vi "zadanie4.vi"() -> ()   [LabVIEW 2019]
uses:
  <vilib>/Utility/file.llb/Write Delimited Spreadsheet (DBL).vi
  <vilib>/ptbypt/NI_PtbyPt.lvlib
panel:
  out "Histogram":dynamicdata(graph)
  out "XY Graph":cluster{"time":dbl[], "value":dbl[]}(graph)
  out "Waveform Chart":cluster{"Numeric":dbl, "mean":dbl}(graph)
  in  "stop":bool
  out "Numeric":dbl
  out "read buffer":string
  in  "Light intensity [%]":dbl(ramp)
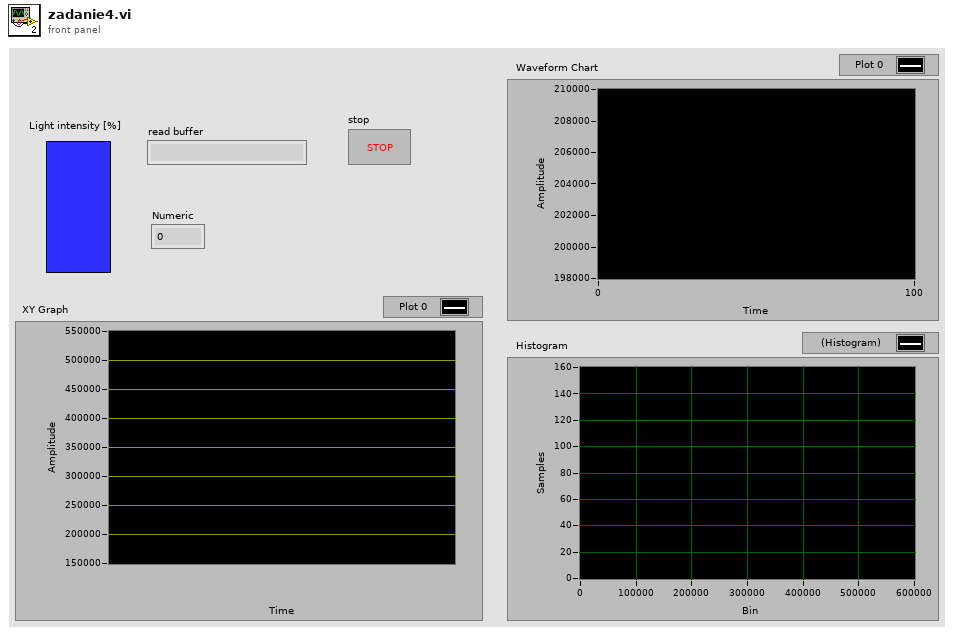
[diagram p1: front panel]
types:
  T1 = enum16{"Configure Port", "Write", "Read", "Close"}
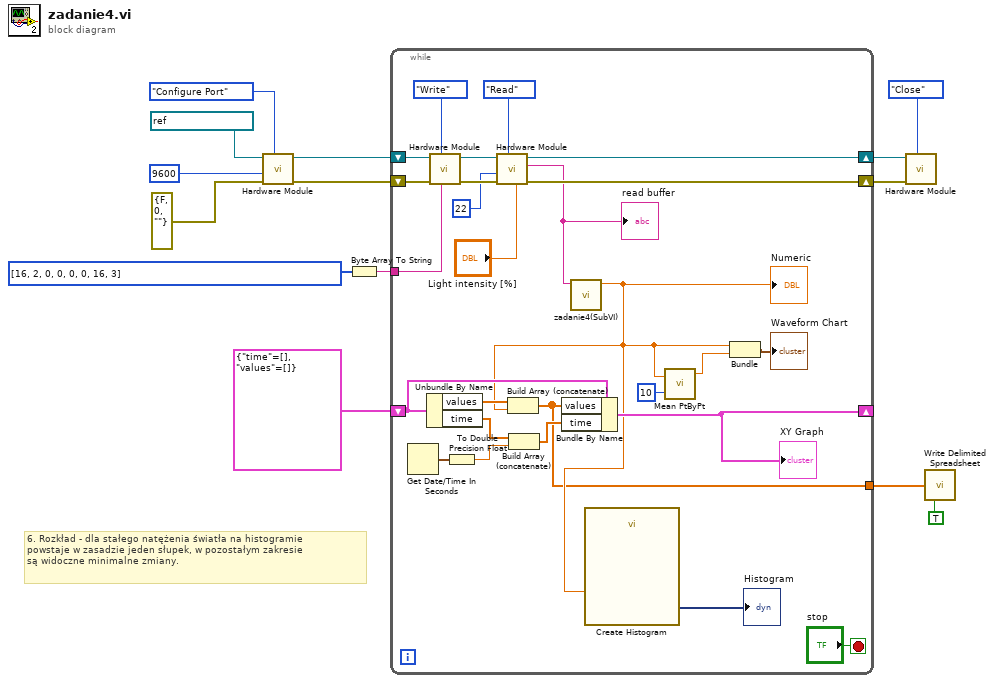
[diagram p0: block diagram]
diagram:
  # "6. Rozkład - dla stałego natężenia światła na histogramie \npowstaje w zasadzie jeden słupek, w pozostałym zakresie \nsą widoczne minimalne zmiany."
  n1 = call "Hardware Module.vi"("State"=T1."Configure Port", "error in (no error)"=errorcluster {"status"=FALSE, "code"=0, "source"=""}, "baud rate (9600)"=u32 9600, "VISA resource name"=refnum<visa-resource-name> "VirtualDevice1") -> ("error out"=w12:errorcluster, "VISA resource name out"=w11:refnum<visa-resource-name>)  [unwired: 4 in, 2 out]
  n2 = Byte Array To String(unsigned byte array=u8[] [16, 2, 0, 0, 0, 0, 16, 3]) -> (string=w4:string)
  n3 = while {
    tunnel: w4 -> [w32]
    shift-right: [w37] -> w13
    shift-left: w12 -> [w36]
    shift-right: [w39] -> w14
    shift-left: w11 -> [w35]
    shift-right: [w21] -> _
    shift-left: cluster{"time":dbl[], "values":dbl[]} {"time"=[], "values"=[]} -> [w27]
    tunnel: [w15] -> w2
    stop <- "stop" stop-if-true
    n4 = Get Date/Time In Seconds() -> (seconds since 1Jan1904=w23:timestamp)
    n5 = Unbundle By Name(w27) -> ("values"=w26:dbl[], "time"=w25:dbl[])
    n6 = call "Hardware Module.vi"("write buffer"=w32, "State"=T1."Write", "error in (no error)"=w36, "VISA resource name"=w35) -> ("error out"=w38:errorcluster, "VISA resource name out"=w40:refnum<visa-resource-name>)  [unwired: 4 in, 2 out]
    n7 = To Double Precision Float(number=w23) -> (double precision float=w22:dbl)
    n8 = call "Hardware Module.vi"("Light intensity [%]"="Light intensity [%]", "State"=T1."Read", "error in (no error)"=w38, "byte count"=u32 22, "VISA resource name"=w40) -> ("error out"=w37:errorcluster, "read buffer"=w29:string, "VISA resource name out"=w39:refnum<visa-resource-name>)  [unwired: 3 in, 1 out]
    "read buffer" <- w29
    n9 = Build Array (concatenate)(w25, w22) -> (w24:dbl[])
    n10 = call "zadanie4(SubVI).vi"("read buffer"=w29) -> ("Numeric"=w17:dbl)  [unwired: 10 in]
    "Numeric" <- w17
    n11 = Build Array (concatenate)(w26, w17) -> (w15:dbl[])
    n12 = Bundle By Name(cluster=w27, "values"=w15, "time"=w24) -> (w21:cluster{"time":dbl[], "values":dbl[]})
    "XY Graph" <- w21
    n13 = call "Create Histogram"("Signal"=w17) -> ("Histogram"=→"Histogram":dynamicdata)  [unwired: 9 in, 1 out]
    n14 = call <vilib>:"Mean PtByPt.vi"("x"=w17, "sample length"=10) -> ("mean"=w18:dbl)  [unwired: 2 in, 1 out]
    n15 = Bundle("Numeric"=w17, "mean"=w18) -> (→"Waveform Chart":cluster{"Numeric":dbl, "mean":dbl})  [unwired: 1 in]
  }
  n16 = call "Hardware Module.vi"("State"=T1."Close", "error in (no error)"=w13, "VISA resource name"=w14) -> ()  [unwired: 5 in, 4 out]
  n17 = call-poly <vilib>:"Write Delimited Spreadsheet.vi"("1D data"=w2, "transpose? (no:F)"=TRUE) -> ()  [unwired: 12 in, 2 out]
